vi "Find.vi"(8 "error in":errorcluster, 11 "target in":refnum<k24>) -> (0 "error out":errorcluster, 2 "data sharing framework custom device":T1 format="%.0x", 3 "target out":refnum<k24>, 4 "found?":bool)   [LabVIEW 2019, in "Data Sharing Framework Custom Device Scripting.lvlib"]
doc: "For the specified <b>target in</b>, finds the node identifier for the instance of the Data Sharing Framework custom device."
uses:
  Data Sharing Framework Custom Device Scripting.lvlib
  NationalInstruments.VeriStand.SystemDefinitionAPI
  <vilib>/NI VeriStand/Custom Device API/Custom Device Item Ref.ctl
  Shared/DSF Shared.lvlib
  <vilib>/NI VeriStand/Custom Device API/Custom Device API.lvlib
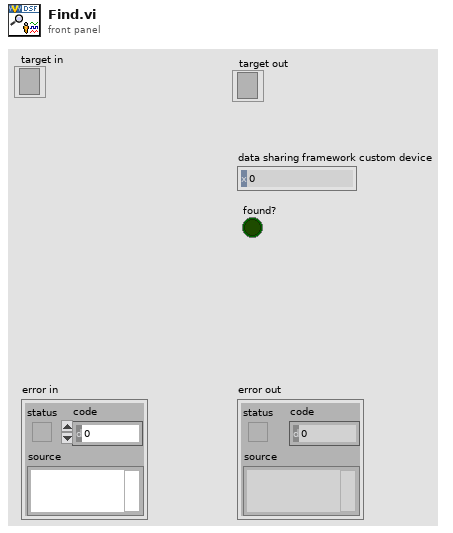
[diagram p1: front panel]
types:
  T1 = typedef "Custom Device API.lvlib/Custom Device Item Ref.ctl" = u64
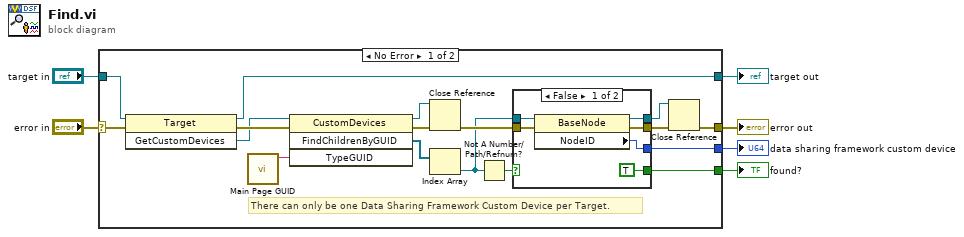
[diagram p0: block diagram]
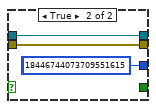
[diagram p2: hidden frame]
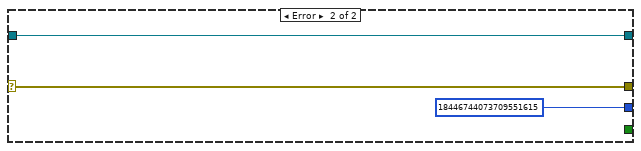
[diagram p3: hidden frame]
diagram:
  n1 = case shown="No Error" "error in" {
    selector: "error in" -> [w23 w35]
    tunnel: [w13 w35] -> w6
    tunnel: "target in" -> [w22 w34]
    tunnel: [w16 w34] -> w3
    tunnel: [w15 u64 18446744073709551615 ("NodeID")] -> w2
    tunnel: [w7 _] -> w1
    frame No Error {
      # "There can only be one Data Sharing Framework Custom Device per Target."
      n2 = invoke class="Target" method="GetCustomDevices"(reference=w22, error in=w23) -> (reference out=w16:refnum<k24>, error out=w21:errorcluster, "GetCustomDevices"=w20:refnum<k24>)  [unwired: 1 in]
      n3 = call "Main Page GUID.vi"() -> ("Main Page GUID"=w9:string)  [unwired: 11 in]
      n4 = invoke class="CustomDevices" method="FindChildrenByGUID"(reference=w20, error in=w21, "TypeGUID"=w9) -> (reference out=w19:refnum<k24>, error out=w18:errorcluster, "FindChildrenByGUID"=w11:refnum<k24>[])  [unwired: 1 in, 1 out]
      n5 = Close Reference(reference=w19, error in (no error)=w18) -> (error out=w17:errorcluster)
      n6 = Index Array(array=w11) -> (element=w10:refnum<k24>)  [unwired: 1 in]
      n7 = Not A Number/Path/Refnum?(number/path/refnum=w10) -> (NaN/Path/Refnum?=w8:bool)
      n8 = case shown="False" w8 {
        tunnel: [w25 w32] -> w12
        tunnel: w17 -> [w27 w32]
        tunnel: w10 -> [w29 w31]
        tunnel: [w28 u64 18446744073709551615 ("NodeID")] -> w15
        tunnel: [w26 w31] -> w14
        tunnel: [TRUE _] -> w7
        frame False {
          n9 = property class="BaseNode"(reference=w29, error in=w27) -> (reference out=w26:refnum<k24>, error out=w25:errorcluster, "NodeID"=w28:u64)
        }
        frame True {
          (unwired) u64 18446744073709551615 ("NodeID")
        }
      }
      n10 = Close Reference(reference=w14, error in (no error)=w12) -> (error out=w13:errorcluster)
    }
    frame Error {
    }
  }
  "target out" <- w3
  "error out" <- w6
  "data sharing framework custom device" <- w2
  "found?" <- w1
